vi "Tx Async.vi"(8 "error in (no error)":errorcluster, 11 "Framework in":refnum<class "Framework.lvclass">) -> (0 "error out":errorcluster, 3 "Framework out":refnum<class "Framework.lvclass">)   [LabVIEW 2017, in "DSF Core.lvlib" / "Framework.lvclass"]
uses:
  Framework.lvclass
  Framework.lvclass/Framework.ctl
  Plugin/Plugin.lvclass
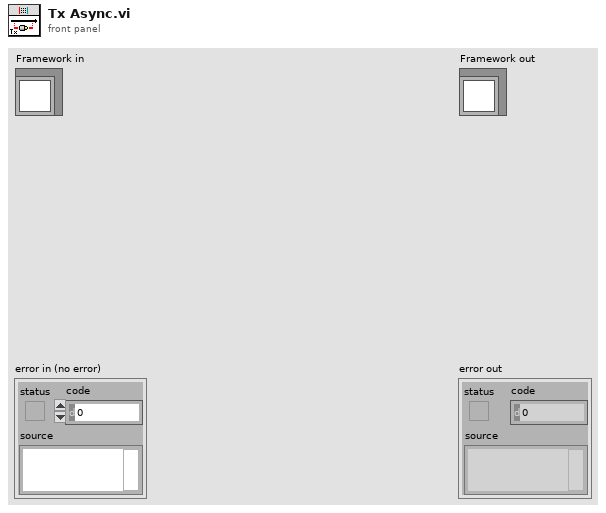
[diagram p1: front panel]
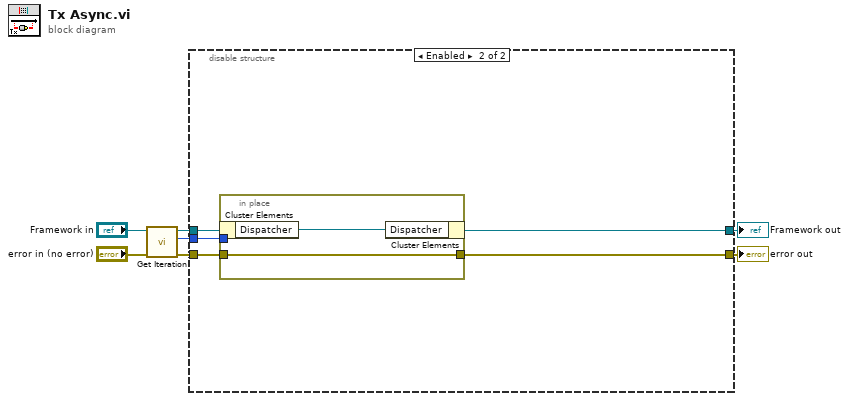
[diagram p0: block diagram]
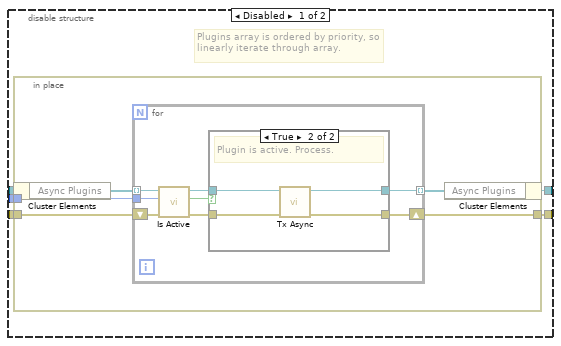
[diagram p2: hidden frame]
diagram:
  n1 = call "Get Iteration.vi"("Framework in"="Framework in") -> ("iteration"=w3:u64, "Framework out"=w1:refnum<class "Framework.lvclass">)  [unwired: 9 in]
  n2 = disable-structure shown="Enabled" {
    disable-tunnel: "error in (no error)" -> [w11 w32]
    disable-tunnel: [w10 w30] -> w5
    disable-tunnel: [w9 w31] -> w4
    disable-tunnel: w3 -> [w8 w33]
    disable-tunnel: w1 -> [w7 w34]
    frame Disabled {
      # "Plugins array is ordered by priority, so linearly iterate through array."
      n3 = in-place {
        in-place-border: w11 -> [w16]
        in-place-border: [w15] -> w10
        in-place-border: w8 -> [w12]
        n4 = in-place-cluster #1(w7) -> ("Async Plugins"=w14:refnum<class "Plugin.lvclass">[])
        n5 = for {
          tunnel: w14 -> [w20] mode=indexing
          tunnel: [w23] -> w13 mode=indexing
          shift-right: [w22] -> w15
          shift-left: w16 -> [w21]
          tunnel: w12 -> [w17]
          n6 = call "Is Active.vi"("cycle count"=w17, "Plugin in"=w20) -> ("active this cycle?"=w18:bool, "Plugin out"=w19:refnum<class "Plugin.lvclass">)  [unwired: 8 in]
          n7 = case shown="True" w18 {
            tunnel: w19 -> [w25 w29]
            tunnel: [w25 w28] -> w23
            tunnel: [w24 w26] -> w22
            tunnel: w21 -> [w24 w27]
            frame False {
              # "Plugin is not active. Skip."
            }
            frame True {
              # "Plugin is active. Process."
              n8 = call "Tx Async.vi"("error in (no error)"=w27, "Plugin in"=w29) -> ("error out"=w26:errorcluster, "Plugin out"=w28:refnum<class "Plugin.lvclass">)  [unwired: 8 in]
            }
          }
        }
        n9 = in-place-cluster #1("Async Plugins"=w13) -> (w9:refnum<class "Framework.lvclass">)
      }
    }
    frame Enabled {
      n10 = in-place {
        in-place-border: w32 -> [w35]
        in-place-border: w33 -> [_]
        in-place-border: [w35] -> w30
        n11 = in-place-cluster #2(w34) -> ("Dispatcher"=w36:refnum<class "Dispatcher.lvclass">)
        n12 = in-place-cluster #2("Dispatcher"=w36) -> (w31:refnum<class "Framework.lvclass">)
      }
    }
  }
  "error out" <- w5
  "Framework out" <- w4
